vi "imaqio_Download.vi"(0 "handle In":T1, 5 "Array":u8[](array[numeric])=array[320146 elements], 11 "error in":errorcluster) -> (4 "handle out":T1, 15 "error out":errorcluster)   [LabVIEW 2017]
uses:
  <vilib>/LabVIEW Targets/FPGA/RIO/nirio_driverPrimitives.llb/_nirio_device_handleType.ctl
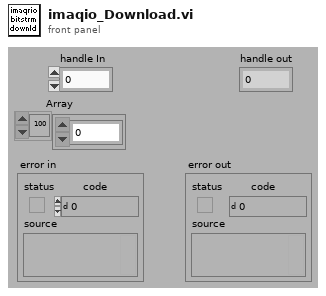
[diagram p1: front panel]
types:
  T1 = typedef "_nirio_device_handleType.ctl" = u32
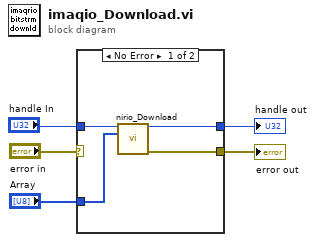
[diagram p0: block diagram]
diagram:
  n1 = case shown="No Error" "error in" {
    selector: "error in" -> [_ w11]
    tunnel: [w7 w11] -> w3
    tunnel: "handle In" -> [w9 w10]
    tunnel: "Array" -> [w8 _]
    tunnel: [w6 w10] -> w2
    frame No Error {
      n2 = call <vilib>:"nirio_Download.vi"("handle in"=w9, "bitstream"=w8) -> ("handle out"=w6:T1, "error out"=w7:errorcluster)  [unwired: 1 in, 11 out]
    }
    frame Error {
    }
  }
  "error out" <- w3
  "handle out" <- w2
